vi "example_microFPGA_camera.vi"() -> ()   [LabVIEW 2021]
panel:
  in  "write or read":u16(ring)=1 items=["read", "write"]
  out "Camera_sw_start_READ":u16(ring)=1 items=["Stop = 0", "Start = 1 "]
  in  "milliseconds to RUN":u32=2000
  out "value write confirm 11":bool=TRUE
  in  "Camera_sw_start_WRITE":u16(ring)=1 items=["Stop = 0", "Start = 1 "]
  out "camera_laser_delay_time_READ":u32(slide)=500 max=65535 step=1 scale=0.0..665535.0 scale format="%u us"
  out "value write confirm 10":bool=TRUE
  in  "camera_laser_delay_time_WRITE":u32(slide)=500 max=65535 step=1 scale=0.0..65535.0 scale format="%u us"
  out "camera_exposure_time_READ":u32(slide)=10000 max=65535 step=1 scale=0.0..1048575.0 scale format="%u us"
  out "value write confirm 9":bool=TRUE
  in  "camera_exposure_time_WRITE":u32(slide)=10000 max=1048580 step=1 scale=0.0..1048575.0 scale format="%u us"
  out "camera_readout_time_READ":u32(slide)=2000 max=65535 step=1 scale=0.0..665535.0 scale format="%u us"
  out "value write confirm 8":bool=TRUE
  in  "camera_readout_time_WRITE":u32(slide)=2000 max=65535 step=1 scale=0.0..65535.0 scale format="%u us"
  out "Camera_mode_READ":u16(ring)=1 items=["Passive = 0", "Active = 1 "]
  in  "Camera_mode_WRITE":u16(ring)=1 items=["Passive = 0", "Active = 1 "]
  out "value write confirm 7":bool=TRUE
  in  "camera_fire_pulse_time_WRITE":u32(slide)=1500 max=65535 step=1 scale=0.0..1048575.0 scale format="%u us"
  out "camera_fire_pulse_time_READ":u32(slide)=1500 max=65535 step=1 scale=0.0..1048575.0 scale format="%u us"
  out "value write confirm 6":bool=TRUE
  out "Version":u16=3
  in  "close Application":bool=TRUE
  in  "send parameters":bool
  # "camera control"
  # "CAMERA"
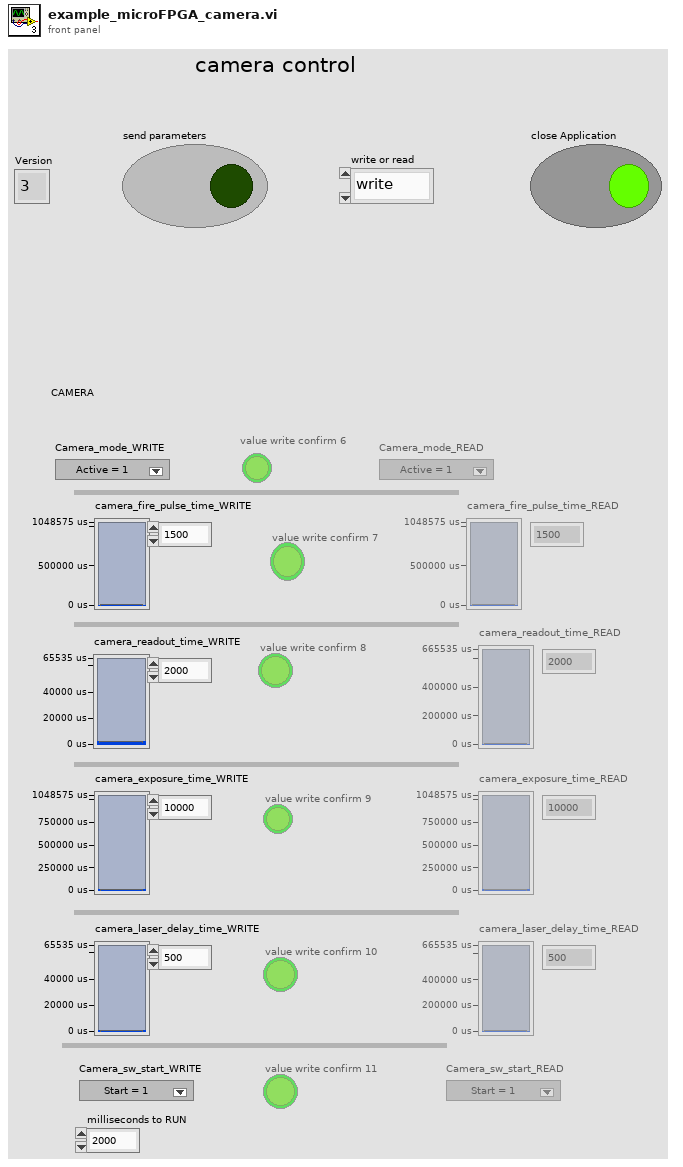
[diagram p1: front panel]
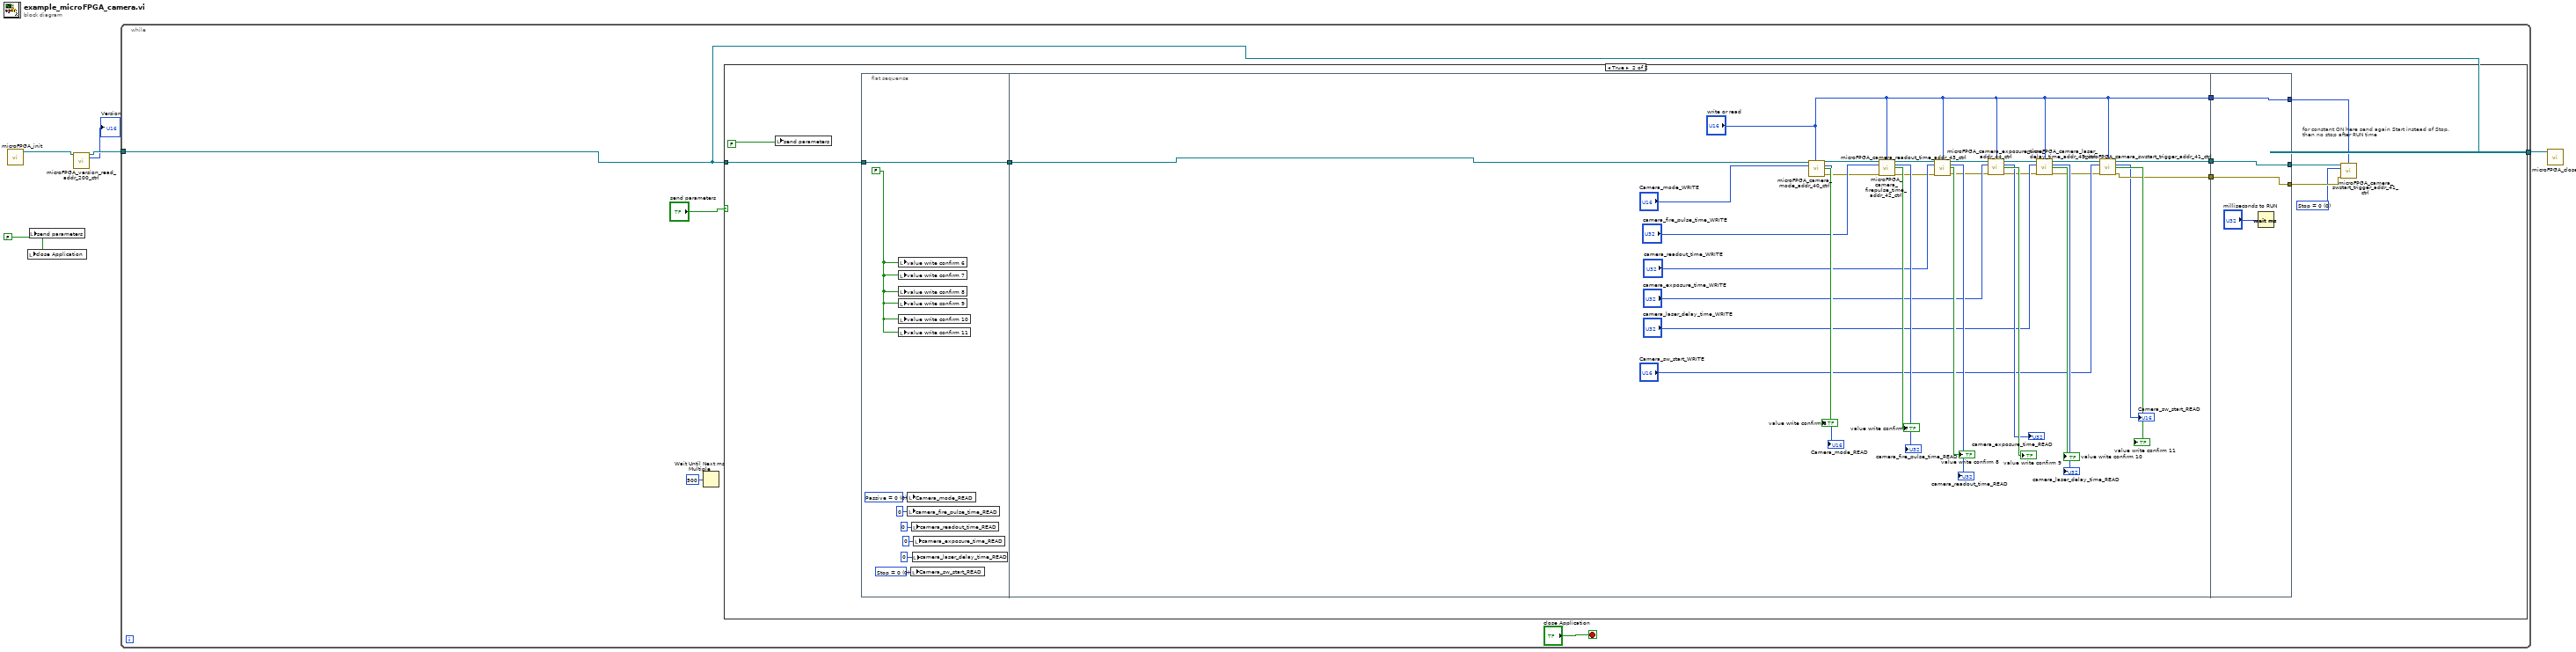
[diagram p0: block diagram]
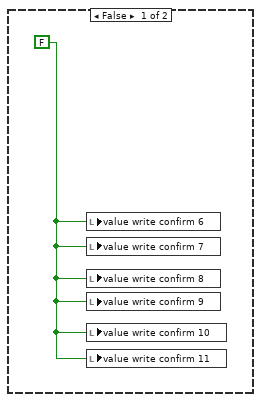
[diagram p2: hidden frame]
diagram:
  w5 = FALSE ("write")
  n1 = call "microFPGA_init.vi"() -> ("VISA resource name out"=w3:refnum<visa-resource-name>)  [unwired: 10 in, 1 out]
  n2 = local write "close Application"(w5) -> ()
  n3 = local write "send parameters"(w5) -> ()
  n4 = call "microFPGA_version_read_addr_200_ctrl.vi"("VISA resource name"=w3) -> ("VISA resource name 2"=w2:refnum<visa-resource-name>, "Version"=→"Version":u16)  [unwired: 12 in, 1 out]
  n5 = while {
    tunnel: w2 -> [w6]
    tunnel: [w6] -> w4
    stop <- "close Application" stop-if-true
    n6 = Wait Until Next ms Multiple(millisecond multiple=u32 500) -> ()  [unwired: 1 out]
    n7 = case shown="True" "send parameters" {
      tunnel: w6 -> [_ w19]
      frame False {
        w10 = FALSE ("value write confirm")
        n8 = local write "value write confirm 6"(w10) -> ()
        n9 = local write "value write confirm 7"(w10) -> ()
        n10 = local write "value write confirm 8"(w10) -> ()
        n11 = local write "value write confirm 9"(w10) -> ()
        n12 = local write "value write confirm 10"(w10) -> ()
        n13 = local write "value write confirm 11"(w10) -> ()
      }
      frame True {
        w11 = u16 0 items=["Stop = 0", "Start = 1 "] ("Camera_sw_start_WRITE 2")
        # "for constant ON here send again Start instead of Stop. \nthen no stop after RUN time"
        n14 = local write "send parameters"(FALSE ("write")) -> ()
        n15 = flat-sequence {
          tunnel: w19 -> [w28]
          tunnel: [w28] -> w12
          tunnel: [w38] -> w17
          tunnel: [w37] -> w16
          tunnel: ["write or read"] -> w14
          tunnel: w12 -> [w29]
          tunnel: [w63] -> w18
          tunnel: w17 -> [w63]
          tunnel: w16 -> [w62]
          tunnel: [w62] -> w15
          tunnel: w14 -> [w61]
          tunnel: [w61] -> w13
          frame #0 {
            w27 = u16 0 items=["Stop = 0", "Start = 1 "] ("Camera_sw_start_READ")
            w22 = u16 0 items=["Passive = 0", "Active = 1 "] ("Camera_mode_READ")
            w21 = FALSE ("value write confirm")
            n16 = local write "value write confirm 6"(w21) -> ()
            n17 = local write "value write confirm 7"(w21) -> ()
            n18 = local write "value write confirm 8"(w21) -> ()
            n19 = local write "value write confirm 9"(w21) -> ()
            n20 = local write "value write confirm 10"(w21) -> ()
            n21 = local write "value write confirm 11"(w21) -> ()
            n22 = local write "Camera_mode_READ"(w22) -> ()
            n23 = local write "camera_fire_pulse_time_READ"(u32 0 ("camera_fire_pulse_time_READ")) -> ()
            n24 = local write "Camera_sw_start_READ"(w27) -> ()
            n25 = local write "camera_readout_time_READ"(u32 0 ("camera_readout_time_READ")) -> ()
            n26 = local write "camera_laser_delay_time_READ"(u32 0 ("camera_laser_delay_time_READ")) -> ()
            n27 = local write "camera_exposure_time_READ"(u32 0 ("camera_exposure_time_READ")) -> ()
          }
          frame #1 {
            n28 = call "microFPGA_camera_mode_addr_40_ctrl.vi"("VISA resource name"=w29, "write or read"="write or read", "Camera_mode_WRITE"="Camera_mode_WRITE") -> ("VISA resource name 2"=w59:refnum<visa-resource-name>, "Camera_mode_READ"=→"Camera_mode_READ":u16, "value write confirm"=→"value write confirm 6":bool, "error out"=w32:errorcluster)  [unwired: 8 in, 1 out]
            n29 = call "microFPGA_camera_firepulse_time_addr_42_ctrl.vi"("VISA resource name"=w59, "write or read"="write or read", "camera_fire_pulse_time_WRITE"="camera_fire_pulse_time_WRITE", "error in (no error)"=w32) -> ("VISA resource name 2"=w50:refnum<visa-resource-name>, "camera_fire_pulse_time_READ"=→"camera_fire_pulse_time_READ":u32, "value write confirm"=→"value write confirm 7":bool, "error out"=w33:errorcluster)  [unwired: 7 in, 1 out]
            n30 = call "microFPGA_camera_readout_time_addr_43_ctrl.vi"("VISA resource name"=w50, "write or read"="write or read", "camera_readout_time_WRITE"="camera_readout_time_WRITE", "error in (no error)"=w33) -> ("VISA resource name 2"=w48:refnum<visa-resource-name>, "camera_readout_time_READ"=→"camera_readout_time_READ":u32, "value write confirm"=→"value write confirm 8":bool, "error out"=w34:errorcluster)  [unwired: 7 in, 1 out]
            n31 = call "microFPGA_camera_exposure_time_addr_44_ctrl.vi"("VISA resource name"=w48, "write or read"="write or read", "camera_exposure_time_WRITE"="camera_exposure_time_WRITE", "error in (no error)"=w34) -> ("VISA resource name 2"=w47:refnum<visa-resource-name>, "camera_exposure_time_READ"=→"camera_exposure_time_READ":u32, "value write confirm"=→"value write confirm 9":bool, "error out"=w35:errorcluster)  [unwired: 7 in, 1 out]
            n32 = call "microFPGA_camera_laser_delay_time_addr_45_ctrl.vi"("VISA resource name"=w47, "write or read"="write or read", "camera_laser_delay_time_WRITE"="camera_laser_delay_time_WRITE", "error in (no error)"=w35) -> ("VISA resource name 2"=w41:refnum<visa-resource-name>, "camera_laser_delay_time_READ"=→"camera_laser_delay_time_READ":u32, "value write confirm"=→"value write confirm 10":bool, "error out"=w36:errorcluster)  [unwired: 7 in, 1 out]
            n33 = call "microFPGA_camera_swstart_trigger_addr_41_ctrl.vi"("VISA resource name"=w41, "write or read"="write or read", "Camera_sw_start_WRITE"="Camera_sw_start_WRITE", "error in (no error)"=w36) -> ("VISA resource name 2"=w38:refnum<visa-resource-name>, "Camera_sw_start_READ"=→"Camera_sw_start_READ":u16, "value write confirm"=→"value write confirm 11":bool, "error out"=w37:errorcluster)  [unwired: 7 in, 1 out]
          }
          frame #2 {
            n34 = Wait (ms)(milliseconds to wait="milliseconds to RUN") -> ()  [unwired: 1 out]
          }
        }
        n35 = call "microFPGA_camera_swstart_trigger_addr_41_ctrl.vi"("VISA resource name"=w18, "write or read"=w13, "Camera_sw_start_WRITE"=w11, "error in (no error)"=w15) -> ()  [unwired: 7 in, 5 out]
      }
    }
  }
  n36 = call "microFPGA_close.vi"("VISA resource name"=w4) -> ()  [unwired: 11 in]
